vi "metadata.update.unit.request.vi"(8 "error in":errorcluster, 10 "Unit":string, 11 "channel in":refnum<class "Channel.lvclass">) -> (0 "error out":errorcluster, 3 "JSON Payload":string)   [LabVIEW 2020, in "Nominal Client.lvclass"]
uses:
  submodules/nominal-streaming-labview-ffi/lv_src/Channel/Channel.lvclass
  submodules/nominal-streaming-labview-ffi/lv_src/Channel/Channel.lvclass/Channel.ctl
  submodules/nominal-streaming-labview-ffi/lv_src/Stream/Stream.lvclass/Stream.ctl
  3536d236-6dd3-40ff-a9be-19a538437cb9.vi
  f593ea07-b612-4092-bdd6-7231a3a1b6a9.vi
  5a4ea93c-afbb-4790-a514-34ee44610bed.vi
  submodules/nominal-streaming-labview-ffi/lv_src/Channel/name.get.vi
  submodules/nominal-streaming-labview-ffi/lv_src/Channel/stream.get.vi
  submodules/nominal-streaming-labview-ffi/lv_src/Stream/datasetRid.get.vi
  <vilib>/JDP Science/JSONtext/Variant to JSON Text.vi
  submodules/nominal-streaming-labview-ffi/lv_src/Stream/Stream.lvclass
  <vilib>/JDP Science/JSONtext/LVClass Serializer/JSONtext LVClass Serializer.lvclass
  Nominal Client/Nominal Client.lvclass
  Nominal Client/Nominal Client.lvclass/Nominal Client.ctl
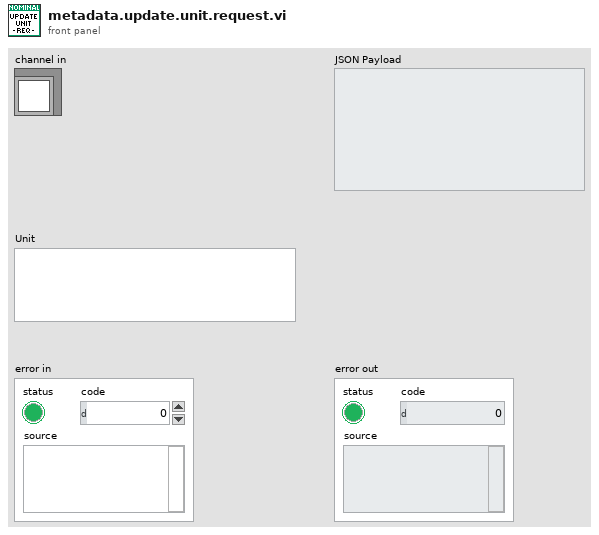
[diagram p1: front panel]
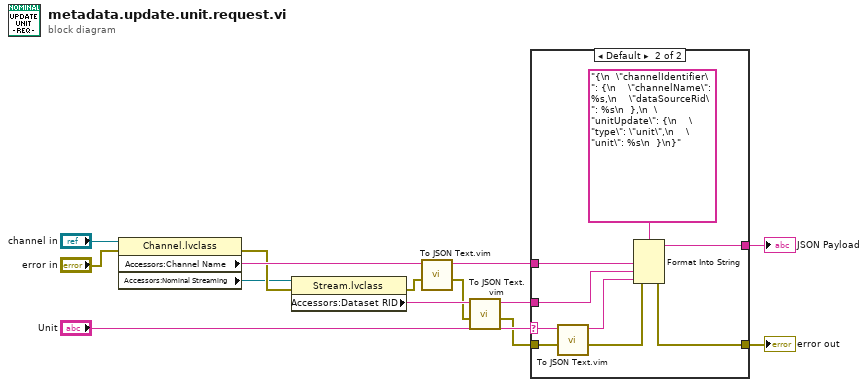
[diagram p0: block diagram]
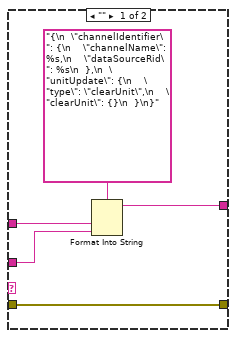
[diagram p2: hidden frame]
diagram:
  n1 = property class="Channel.lvclass"(reference="channel in", error in="error in") -> (error out=w12:errorcluster, "Accessors:Channel Name"=w13:string, "Accessors:Nominal Streaming"=w6:refnum<class "Stream.lvclass">)  [unwired: 1 out]
  n2 = property class="Stream.lvclass"(reference=w6, error in=w12) -> (error out=w8:errorcluster, "Accessors:Dataset RID"=w3:string)  [unwired: 1 out]
  n3 = call "To JSON Text.vim"("error in (no error)"=w8, "Anything"=w13) -> ("error out"=w1:errorcluster, "<JSON>"=w7:string)  [unwired: 8 in]
  n4 = call "To JSON Text.vim"("error in (no error)"=w1, "Anything"=w3) -> ("error out"=w4:errorcluster, "<JSON>"=w2:string)  [unwired: 8 in]
  n5 = case shown="Default" "Unit" {
    selector: "Unit" -> [_ w24]
    tunnel: [w17 w27] -> w11
    tunnel: [w19 w26] -> w10
    tunnel: w7 -> [w18 w25]
    tunnel: w4 -> [w19 w23]
    tunnel: w2 -> [w16 w20]
    frame "" {
      n6 = Format Into String(format string="{\n  \"channelIdentifier\": {\n    \"channelName\": %s,\n    \"dataSourceRid\": %s\n  },\n  \"unitUpdate\": {\n    \"type\": \"clearUnit\",\n    \"clearUnit\": {}\n  }\n}", w18, w16) -> (resulting string=w17:string)  [unwired: 2 in, 1 out]
    }
    frame Default {
      n7 = call "To JSON Text.vim"("error in (no error)"=w23, "Anything"=w24) -> ("error out"=w21:errorcluster, "<JSON>"=w22:string)  [unwired: 8 in]
      n8 = Format Into String(format string="{\n  \"channelIdentifier\": {\n    \"channelName\": %s,\n    \"dataSourceRid\": %s\n  },\n  \"unitUpdate\": {\n    \"type\": \"unit\",\n    \"unit\": %s\n  }\n}", error in=w21, w25, w20, w22) -> (resulting string=w27:string, error out=w26:errorcluster)  [unwired: 1 in]
    }
  }
  "error out" <- w10
  "JSON Payload" <- w11
